vi "calc_images_for_display.vi"(6 "Raw data in":dbl[][][](array[numeric]), 7 "Lower bounds array":dbl[](array[numeric]), 8 "error in":errorcluster, 9 "Color tables display":T2[](array[typedef])=[enum."Grayscale"], 10 "Upper bounds array":dbl[](array[numeric]), 11 "Image in":T1) -> (0 "error out":errorcluster, 3 "Image Out":T1)   [LabVIEW 2011, in "Fiberscope_library.lvlib"]
uses:
  Fiberscope_library.lvlib
  typedefs/color_palette_enum.ctl
  <vilib>/vision/Image Controls.llb/IMAQ Image.ctl
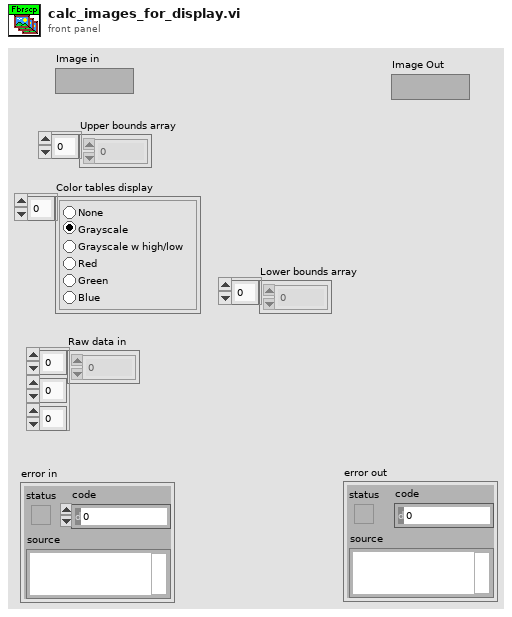
[diagram p1: front panel]
types:
  T1 = typedef "IMAQ Image.ctl" = refnum<image>
  T2 = typedef "Fiberscope_library.lvlib/color_palette_enum.ctl" = enum32{"None", "Grayscale", "Grayscale w high/low", "Red", "Green", "Blue"}
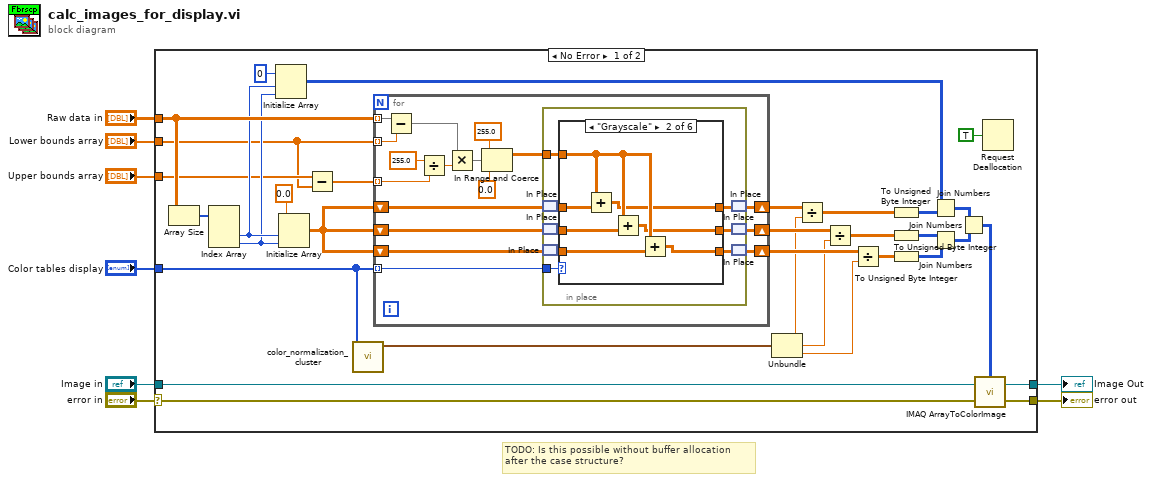
[diagram p0: block diagram]
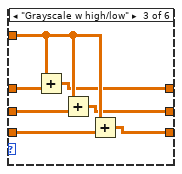
[diagram p3: hidden frame]
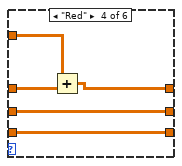
[diagram p4: hidden frame]
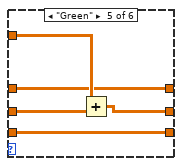
[diagram p5: hidden frame]
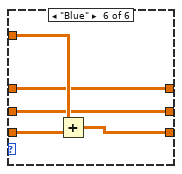
[diagram p6: hidden frame]
diagram:
  # "TODO: Is this possible without buffer allocation\nafter the case structure?"
  n1 = case shown="No Error" "error in" {
    selector: "error in" -> [w14 w99]
    tunnel: "Raw data in" -> [w39 _]
    tunnel: "Image in" -> [w41 w100]
    tunnel: [w40 w100] -> w6
    tunnel: [w13 w99] -> w4
    tunnel: "Upper bounds array" -> [w11 _]
    tunnel: "Color tables display" -> [w35 _]
    tunnel: "Lower bounds array" -> [w10 _]
    frame No Error {
      n2 = Array Size(array=w39) -> (size(s)=w38:i32[])
      n3 = Index Array(array=w38) -> (element #2=w19:i32, element #3=w18:i32)  [unwired: 3 in, 1 out]
      n4 = Initialize Array(u8 0 ("element"), w19, w18) -> (w16:u8[][])
      n5 = Initialize Array(0.0 ("element"), w19, w18) -> (w36:dbl[][])
      n6 = Subtract(x=w11, y=w10) -> (x-y=w9:dbl[])
      n7 = call "color_normalization_cluster.vi"("Color tables array"=w35) -> ("Normalization cluster"=w31:cluster{"[0]":dbl, "[1]":dbl, "[2]":dbl})  [unwired: 10 in]
      n8 = for {
        tunnel: w39 -> [w51] mode=indexing
        tunnel: w35 -> [w58] mode=indexing
        shift-right: [w54] -> w34
        shift-left: w36 -> [w55]
        shift-right: [w53] -> w33
        shift-left: w36 -> [w56]
        shift-right: [w52] -> w32
        shift-left: w36 -> [w57]
        tunnel: w10 -> [w50] mode=indexing
        tunnel: w9 -> [w47] mode=indexing
        n9 = Subtract(x=w51, y=w50) -> (x-y=w46:dbl[][])
        n10 = Divide(x=255.0, y=w47) -> (x/y=w48:dbl)
        n11 = Multiply(x=w46, y=w48) -> (x*y=w45:dbl[][])
        n12 = In Range and Coerce(upper limit=255.0 ("element"), x=w45, lower limit=0.0 ("element")) -> (coerced(x)=w44:dbl[][])  [unwired: 1 out]
        n13 = in-place {
          in-place-border: w58 -> [w66]
          in-place-border: w44 -> [w65]
          n14 = in-place-match #1(w55) -> (w64:dbl[][])
          n15 = in-place-match #2(w56) -> (w63:dbl[][])
          n16 = in-place-match #3(w57) -> (w62:dbl[][])
          n17 = case shown="\"Grayscale\"" w66 {
            tunnel: w65 -> [_ w73 w80 w87 w92 w96]
            tunnel: w64 -> [w69 w76 w83 w88 w90 w94]
            tunnel: w63 -> [w68 w75 w82 w85 w93 w95]
            tunnel: w62 -> [w67 w74 w81 w84 w89 w98]
            tunnel: [w67 w72 w79 w84 w89 w97] -> w61
            tunnel: [w68 w71 w78 w85 w91 w95] -> w60
            tunnel: [w69 w70 w77 w86 w90 w94] -> w59
            frame "None", Default {
            }
            frame "Grayscale" {
              n18 = Add(x=w73, y=w76) -> (x+y=w70:dbl[][])
              n19 = Add(x=w73, y=w75) -> (x+y=w71:dbl[][])
              n20 = Add(x=w73, y=w74) -> (x+y=w72:dbl[][])
            }
            frame "Grayscale w high/low" {
              n21 = Add(x=w80, y=w83) -> (x+y=w77:dbl[][])
              n22 = Add(x=w80, y=w82) -> (x+y=w78:dbl[][])
              n23 = Add(x=w80, y=w81) -> (x+y=w79:dbl[][])
            }
            frame "Red" {
              n24 = Add(x=w87, y=w88) -> (x+y=w86:dbl[][])
            }
            frame "Green" {
              n25 = Add(x=w92, y=w93) -> (x+y=w91:dbl[][])
            }
            frame "Blue" {
              n26 = Add(x=w96, y=w98) -> (x+y=w97:dbl[][])
            }
          }
          n27 = in-place-match #1(w59) -> (w54:dbl[][])
          n28 = in-place-match #2(w60) -> (w53:dbl[][])
          n29 = in-place-match #3(w61) -> (w52:dbl[][])
        }
      }
      n30 = Unbundle(w31) -> ("[0]"=w30:dbl, "[1]"=w29:dbl, "[2]"=w28:dbl)
      n31 = Divide(x=w34, y=w30) -> (x/y=w25:dbl[][])
      n32 = Divide(x=w33, y=w29) -> (x/y=w26:dbl[][])
      n33 = Divide(x=w32, y=w28) -> (x/y=w27:dbl[][])
      n34 = To Unsigned Byte Integer(number=w25) -> (unsigned 8bit integer=w22:u8[][])
      n35 = To Unsigned Byte Integer(number=w26) -> (unsigned 8bit integer=w21:u8[][])
      n36 = To Unsigned Byte Integer(number=w27) -> (unsigned 8bit integer=w20:u8[][])
      n37 = Join Numbers(hi=w16, lo=w22) -> ((hi.lo)=w23:u16[][])
      n38 = Join Numbers(hi=w21, lo=w20) -> ((hi.lo)=w24:u16[][])
      n39 = Join Numbers(hi=w23, lo=w24) -> ((hi.lo)=w15:u32[][])
      n40 = call "IMAQ ArrayToColorImage"("Image Pixels (U32)"=w15, "Image"=w41, "error in (no error)"=w14) -> ("Image Out"=w40:T1, "error out"=w13:errorcluster)  [unwired: 2 in]
      n41 = Request Deallocation(TRUE ("flag")) -> ()
    }
    frame Error {
    }
  }
  "Image Out" <- w6
  "error out" <- w4
